vi "Connection String.vi"(8 "error in (no error)":errorcluster, 10 "FileName":string(combo)="Parameters.db", 11 "SQLite in":refnum<class "SQLite.lvclass">) -> (0 "error out":errorcluster, 2 "String":string, 3 "SQLite out":refnum<class "SQLite.lvclass">)   [LabVIEW 2017, in "SQLite.lvclass"]
doc: "SQL 2008: is connection string\nSQLite: open file path\nMySQL: connection string"
uses:
  SQLite.lvclass
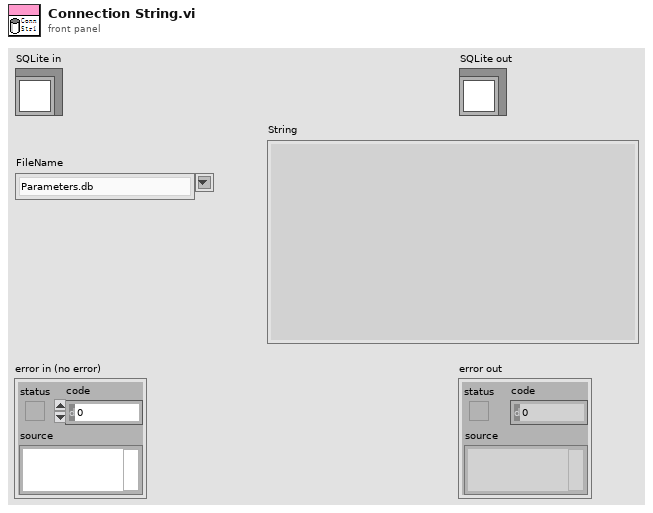
[diagram p1: front panel]
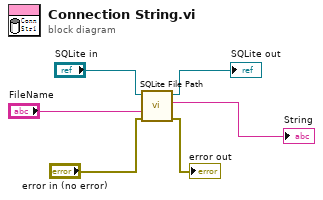
[diagram p0: block diagram]
diagram:
  n1 = call "SQLite File Path.vi"("error in (no error)"="error in (no error)", "SQLiteFileName"="FileName", "SQLite in"="SQLite in") -> ("error out"=→"error out":errorcluster, "string"=→"String":string, "SQLite out"=→"SQLite out":refnum<class "SQLite.lvclass">)  [unwired: 6 in]
